vi "VALEW_Sensors_Hall.vi"(0 "GEA2 Reference In":refnum<k24>, 1 "Gear Multiplier":dbl=0.38125 format="%#_13g", 2 "Gear Ratio":dbl=1.90625 format="%#_13g", 5 "GEA Inputs":T1={"Source"=228, "Destination"=35} {"Destination" format="%.0x"; "Source" format="%.0x"}, 7 "DAQmx Physical Channel":tag="9401_1/ctr2", 9 "Counter Terminal":tag="/9401_1/PFI4", 11 "Error In":errorcluster, 12 "Basket Test RPMs":dbl[](array[numeric])=[125.0, 450.0, 700.0], 13 "Max Error (RPM)":dbl=45.0, 14 "Standalone?":bool) -> (4 "GEA2 Reference Out":refnum<k24>, 6 "Pass/Fail?":bool, 8 "Report Text":string="Shaft RPM253.906250 was found to be 133.000000 and was supposed to be between 122.000000 and 128.000000.  Shaft RPM914.062500 was found to be 479.000000 and was supposed to be between 447.000000 and 453.000000.  Shaft RPM1421.875000 was found to be 745.000000 and was supposed to be between 697.000000 and 703.000000.  ", 15 "Error Out":errorcluster)   [LabVIEW 2016, in "TL27.lvlib"]
doc: "This VI outputs the Test RPMs by generating a frequency that is 0.3 * Test RPM Value and verifies the Basket speed ERD is within the Max Error defined."
uses:
  Projects/TL27.lvlib
  C:/Automation/DLLs/PC Dot Net/GeaCommunication.dll
  Common/LabVIEW GEA2 Toolkit/LabVIEW_GEA2_Toolkit.lvlibp/type defs/Source_Destination.ctl
  Common/LabVIEW GEA2 Toolkit/LabVIEW_GEA2_Toolkit.lvlibp/type defs/ERD Read Data In.ctl
  Common/LabVIEW GEA2 Toolkit/LabVIEW_GEA2_Toolkit.lvlibp/type defs/Data Type.ctl
  <vilib>/DAQmx/create/channels.llb/DAQmx Create Channel (CO-Pulse Generation-Frequency).vi
  <vilib>/DAQmx/configure/timing.llb/DAQmx Timing (Implicit).vi
  Common/LabVIEW GEA2 Toolkit/LabVIEW_GEA2_Toolkit.lvlibp
  <resource>/objmgr/daqmx.rc
panel:
  out "Lim_U_Basket Speed RPM":dbl[](array[numeric])=[128.0, 453.0, 703.0]
  out "Lim_L_Basket Speed RPM":dbl[](array[numeric])=[122.0, 447.0, 697.0]
  out "Basket Speed RPM":dbl[](array[numeric])=[133.0, 479.0, 745.0]
  out "Lim_L_Shaft Speed RPM":dbl[](array[numeric])=[250.90625, 911.0625, 1418.875]
  out "Lim_U_Shaft Speed RPM":dbl[](array[numeric])=[256.90625, 917.0625, 1424.875]
  out "Shaft Speed RPM":dbl[](array[numeric])=[254.0, 914.0, 1422.0]
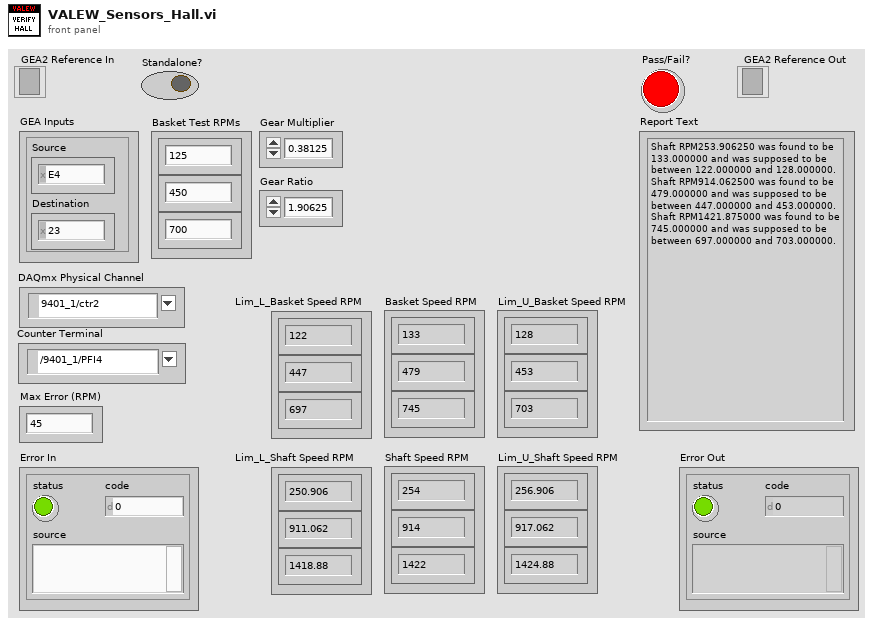
[diagram p1: front panel]
types:
  T1 = typedef "LabVIEW_GEA2_Toolkit.lvlibp/Source_Destination.ctl" = cluster{"Source":u8, "Destination":u8}
  T2 = typedef "LabVIEW_GEA2_Toolkit.lvlibp/ERD Read Data In.ctl" = cluster{"ERD Number":u16, "Data Type":T3}
  T3 = typedef "LabVIEW_GEA2_Toolkit.lvlibp/Data Type.ctl" = enum16{"string", "boolean", "uint8_t", "uint16_t", "uint32_t", "uint64_t", "int8_t", "int16_t", "int32_t", "int64_t"}
  T4 = typedef "LabVIEW_GEA2_Toolkit.lvlibp/ERD Read Data Out.ctl" = cluster{"ERD Number":u16, "Data":string}
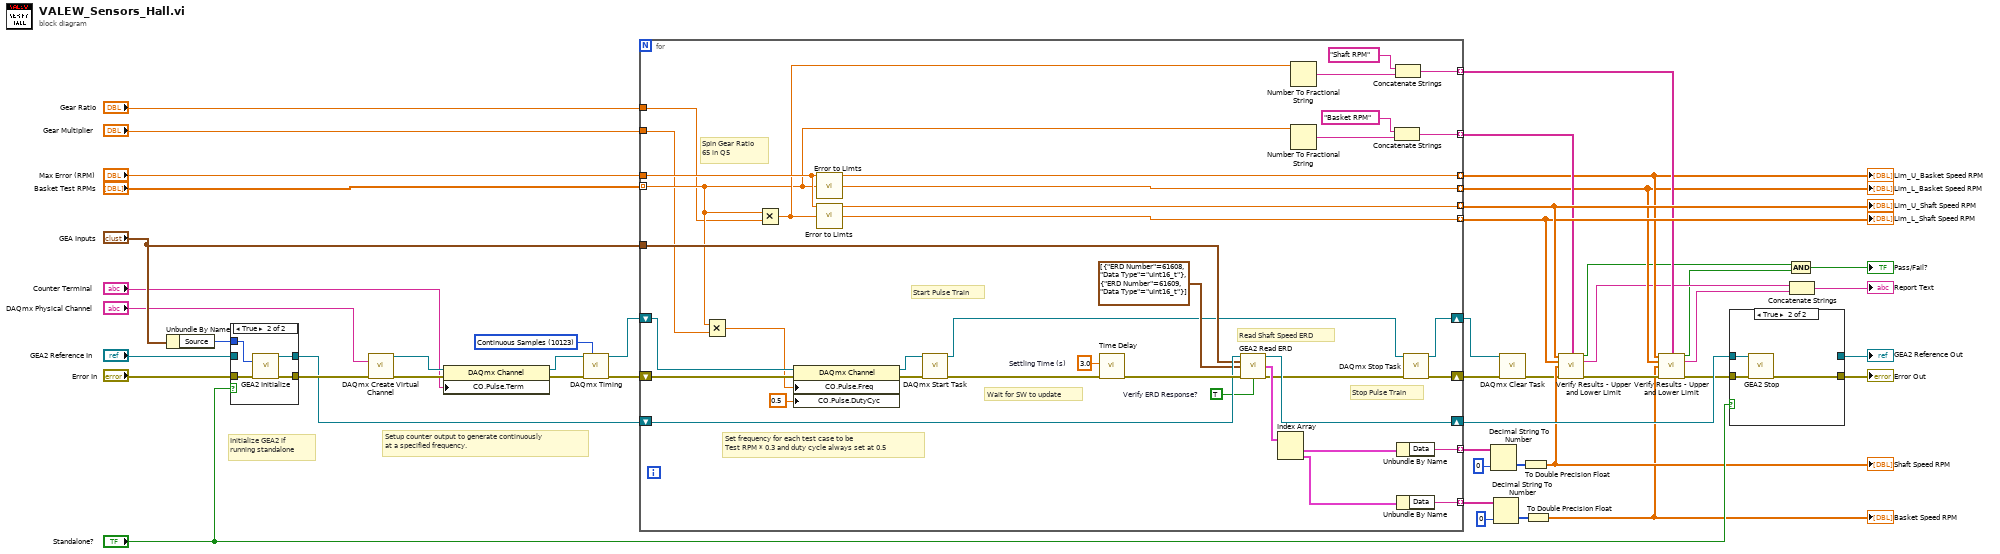
[diagram p0: block diagram]
diagram:
  w28 = 10123 items=["Finite Samples"=10178, "Continuous Samples"=10123, "Hardware Timed Single Point"=12522] ("sample mode")
  # "Setup counter output to generate continuously\nat a specified frequency."
  # "Initialize GEA2 if\nrunning standalone"
  n1 = Unbundle By Name("GEA Inputs") -> ("Source"=w40:u8)
  n2 = case shown="True" "Standalone?" {
    tunnel: "Error In" -> [w50 w54]
    tunnel: [w50 w53] -> w46
    tunnel: "GEA2 Reference In" -> [w49 _]
    tunnel: [w49 w52] -> w42
    tunnel: w40 -> [_ w51]
    frame False {
    }
    frame True {
      n3 = call "GEA2 Initialize.vi"("Source Address"=w51, "error in"=w54) -> ("GEA2 Reference Out"=w52:refnum<k24>, "error out"=w53:errorcluster)  [unwired: 11 in, 1 out]
    }
  }
  n4 = call-poly <vilib>:"DAQmx Create Virtual Channel.vi"("counter"="DAQmx Physical Channel", "error in"=w46) -> ("task out"=w33:refnum<k21>, "error out"=w34:errorcluster)  [unwired: 12 in]
  n5 = property class="DAQmx Channel"(reference=w33, error in=w34, "CO.Pulse.Term"="Counter Terminal") -> (reference out=w29:refnum<k21>, error out=w26:errorcluster)
  n6 = call-poly <vilib>:"DAQmx Timing.vi"("task/channels in"=w29, "sample mode"=w28, "error in"=w26) -> ("task out"=w27:refnum<k21>, "error out"=w25:errorcluster)  [unwired: 11 in]
  n7 = for {
    shift-right: [w81] -> w41
    shift-left: w42 -> [w90]
    shift-right: [w75] -> w45
    shift-left: w27 -> [w84]
    shift-right: [w76] -> w4
    shift-left: w25 -> [w83]
    tunnel: "GEA Inputs" -> [w89]
    tunnel: [w86] -> w38 mode=indexing
    tunnel: "Basket Test RPMs" -> [w57] mode=indexing
    tunnel: "Max Error (RPM)" -> [w64]
    tunnel: [w74] -> w22 mode=indexing
    tunnel: [w73] -> w23 mode=indexing
    tunnel: [w70] -> w20 mode=indexing
    tunnel: [w66] -> w14 mode=indexing
    tunnel: [w65] -> w13 mode=indexing
    tunnel: [w62] -> w17 mode=indexing
    tunnel: [w59] -> w15 mode=indexing
    tunnel: "Gear Multiplier" -> [w56]
    tunnel: "Gear Ratio" -> [w55]
    w85 = TRUE  # Verify ERD Response?
    w92 = 3.0  # Settling Time (s)
    # "Spin Gear Ratio\n65 in Q5"
    # "Stop Pulse Train"
    # "Read Shaft Speed ERD"
    # "Wait for SW to update"
    # "Start Pulse Train"
    # "Set frequency for each test case to be\nTest RPM * 0.3 and duty cycle always set at 0.5"
    n8 = Multiply(x=w57, y=w56) -> (x*y=w67:dbl)
    n9 = Multiply(x=w57, y=w55) -> (x*y=w58:dbl)
    n10 = property class="DAQmx Channel"(reference=w84, error in=w83, "CO.Pulse.Freq"=w67, "CO.Pulse.DutyCyc"=0.5) -> (reference out=w78:refnum<k21>, error out=w79:errorcluster)
    n11 = call "Error to Limts.vi"("Error"=w64, "Value"=w57) -> ("Upper Limit"=w66:dbl, "Lower Limit"=w65:dbl)  [unwired: 12 in]
    n12 = call "Error to Limts.vi"("Error"=w64, "Value"=w58) -> ("Upper Limit"=w73:dbl, "Lower Limit"=w74:dbl)  [unwired: 12 in]
    n13 = call <vilib>:"DAQmx Start Task.vi"("task/channels in"=w78, "error in"=w79) -> ("task out"=w68:refnum<k21>, "error out"=w82:errorcluster)  [unwired: 12 in]
    n14 = call "Time Delay"("error in (no error)"=w82, "Delay Time (s)"=w92) -> ("error out"=w91:errorcluster)  [unwired: 9 in]
    n15 = call "GEA2 Read ERD.vi"("GEA2 Reference In"=w90, "GEA Inputs"=w89, "Read ERD List"=T2[] [{"ERD Number"=61608, "Data Type"=enum."uint16_t"}, {"ERD Number"=61609, "Data Type"=enum."uint16_t"}], "Error In"=w91, "Verify ERD Response?"=w85) -> ("GEA2 Reference Out"=w81:refnum<k24>, "ERD Data Out"=w88:T4[], "Error Out"=w77:errorcluster)  [unwired: 7 in, 1 out]
    n16 = Index Array(array=w88) -> (element #1=w87:T4, element #2=w63:T4)  [unwired: 2 in]
    n17 = Number To Fractional String(number=w58) -> (F-format string=w61:string)  [unwired: 3 in]
    n18 = Number To Fractional String(number=w57) -> (F-format string=w71:string)  [unwired: 3 in]
    n19 = Concatenate Strings("Basket RPM", w71) -> (w70:string)
    n20 = Concatenate Strings("Shaft RPM", w61) -> (w59:string)
    n21 = Unbundle By Name(w87) -> ("Data"=w86:string)
    n22 = Unbundle By Name(w63) -> ("Data"=w62:string)
    n23 = call <vilib>:"DAQmx Stop Task.vi"("task/channels in"=w68, "error in"=w77) -> ("task out"=w75:refnum<k21>, "error out"=w76:errorcluster)  [unwired: 12 in]
  }
  "Lim_U_Shaft Speed RPM" <- w23
  "Lim_L_Shaft Speed RPM" <- w22
  "Lim_U_Basket Speed RPM" <- w14
  "Lim_L_Basket Speed RPM" <- w13
  n24 = Decimal String To Number(string=w38, default (0L)=u16 0 ("default (0 I32)")) -> (number=w36:u16[])  [unwired: 1 in, 1 out]
  n25 = Decimal String To Number(string=w17, default (0L)=u16 0 ("default (0 I32)")) -> (number=w19:u16[])  [unwired: 1 in, 1 out]
  n26 = call <vilib>:"DAQmx Clear Task.vi"("task in"=w45, "error in"=w4) -> ("error out"=w5:errorcluster)  [unwired: 13 in]
  n27 = To Double Precision Float(number=w36) -> (double precision float=w21:dbl[])
  "Shaft Speed RPM" <- w21
  n28 = To Double Precision Float(number=w19) -> (double precision float=w12:dbl[])
  "Basket Speed RPM" <- w12
  n29 = call "Verify Results - Upper and Lower Limit.vi"("Upper Limits"=w23, "Array of Names"=w20, "Lower Limits"=w22, "Results"=w21, "Error In"=w5) -> ("Pass/Fail?"=w8:bool, "Report Text"=w10:string, "Error Out"=w16:errorcluster)  [unwired: 7 in, 1 out]
  n30 = call "Verify Results - Upper and Lower Limit.vi"("Upper Limits"=w14, "Array of Names"=w15, "Lower Limits"=w13, "Results"=w12, "Error In"=w16) -> ("Pass/Fail?"=w7:bool, "Report Text"=w9:string, "Error Out"=w3:errorcluster)  [unwired: 7 in, 1 out]
  n31 = case shown="True" "Standalone?" {
    tunnel: [w93 w97] -> w43
    tunnel: w41 -> [w94 w95]
    tunnel: [w94 _] -> w44
    tunnel: w3 -> [w93 w96]
    frame False {
    }
    frame True {
      n32 = call "GEA2 Stop.vi"("GEA2 Reference In"=w95, "Error In"=w96) -> ("Error Out"=w97:errorcluster)  [unwired: 13 in]
    }
  }
  "Error Out" <- w43
  "GEA2 Reference Out" <- w44
  n33 = And(x=w8, y=w7) -> (x .and. y?=→"Pass/Fail?":bool)
  n34 = Concatenate Strings(w10, w9) -> (→"Report Text":string)
